vi "Populate Names.vi"(10 "Final  Output In":T1={"A-1,  1"="Main", "A-3,  2"="Main", "A-4, 3"="Recircirculation", "A-5, 4"="Scrubber", "A-7, 5"="Oxygen", "A-8, 6"="Vent", "B-1,  7"="Boost A", "B-3, 8"="Boost A", "B-4,  9"="Recircirculation", "B-5, 10"="Scrubber", "B-8, 11"="Vent", "C-1, 12"="Boost B", "C-3, 13"="Boost B", "C-4, 14"="Recircirculation", "C-5,  15"="Scrubber", "C-8, 16"="Vent", "D-1, 17"="Main", "D-3, 18"="Boost A", "D-4,  19"="Boost B", "D-5,  20"="Vent", "D-8,  21"="Vent 2", "B-7"="Oxygen", "C-7"="Oxygen", "D-7"="Oxygen", "A-1"=FALSE, "A-3"=FALSE, "A-4"=FALSE, "A-5"=FALSE, "A-7"=FALSE, "A-8"=FALSE, "B-1"=FALSE, "B-3"=FALSE, "B-4"=FALSE, "B-5"=FALSE, "B-7"=FALSE, "B-8"=FALSE, "C-1"=FALSE, "C-3"=FALSE, "C-4"=FALSE, "C-5"=FALSE, "C-7"=FALSE, "C-8"=FALSE, "D-1"=FALSE, "D-3"=FALSE, "D-4"=FALSE, "D-5"=FALSE, "D-7"=FALSE, "D-8"=FALSE}, 11 "Final Names":T2={"A-1, 1"="Main", "A-3, 2"="Main", "A-4, 3"="Recircirculation", "A-5, 4"="Scrubber", "A-7, 5"="Oxygen", "A-8, 6"="Vent", "B-1,  7"="Boost A", "B-3, 8"="Boost A", "B-4, 9"="Recircirculation", "B-5, 10"="Scrubber", "B-8, 11"="Vent", "C-1, 12"="Boost B", "C-3, 13"="Boost B", "C-4, 14"="Recircirculation", "C-5,  15"="Scrubber", "C-8, 16"="Vent", "D-1, 17"="Main", "D-3, 18"="Boost A", "D-4,  19"="Boost B", "D-5,  20"="Vent", "D-8,  21"="Vent 2"}) -> (3 "Final  Output Out":T1={"A-1,  1"="Main", "A-3,  2"="Main", "A-4, 3"="Recircirculation", "A-5, 4"="Scrubber", "A-7, 5"="Oxygen", "A-8, 6"="Vent", "B-1,  7"="Boost A", "B-3, 8"="Boost A", "B-4,  9"="Recircirculation", "B-5, 10"="Scrubber", "B-8, 11"="Vent", "C-1, 12"="Boost B", "C-3, 13"="Boost B", "C-4, 14"="Recircirculation", "C-5,  15"="Scrubber", "C-8, 16"="Vent", "D-1, 17"="Main", "D-3, 18"="Boost A", "D-4,  19"="Boost B", "D-5,  20"="Vent", "D-8,  21"="Vent 2", "B-7"="Oxygen", "C-7"="Oxygen", "D-7"="Oxygen", "A-1"=FALSE, "A-3"=FALSE, "A-4"=FALSE, "A-5"=FALSE, "A-7"=FALSE, "A-8"=FALSE, "B-1"=FALSE, "B-3"=FALSE, "B-4"=FALSE, "B-5"=FALSE, "B-7"=FALSE, "B-8"=FALSE, "C-1"=FALSE, "C-3"=FALSE, "C-4"=FALSE, "C-5"=FALSE, "C-7"=FALSE, "C-8"=FALSE, "D-1"=FALSE, "D-3"=FALSE, "D-4"=FALSE, "D-5"=FALSE, "D-7"=FALSE, "D-8"=FALSE})   [LabVIEW 2013]
doc: "Populate the names field on the boolean output indicator control."
uses:
  Type Defs/Named Final Output name list ordered.ctl
  Type Defs/Named Final Output name list with 02.ctl
panel:
  # "Channel A"
  # "Channel B"
  # "Channel C"
  # "Channel D"
  # "Channel A"
  # "Channel B"
  # "Channel C"
  # "Channel D"
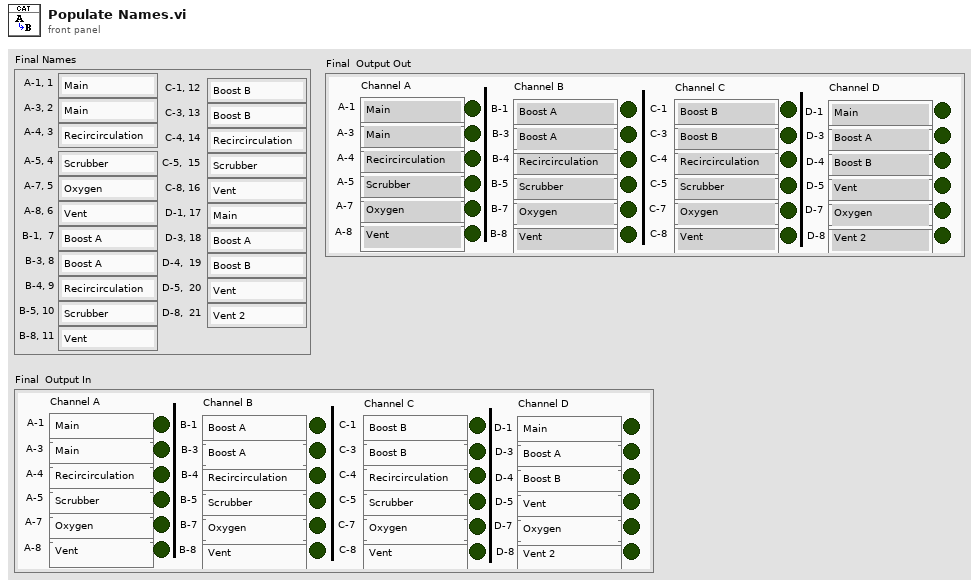
[diagram p1: front panel]
types:
  T1 = typedef "Named Final Output name list with 02.ctl" = cluster{"A-1,  1":string, "A-3,  2":string, "A-4, 3":string, "A-5, 4":string, "A-7, 5":string, "A-8, 6":string, "B-1,  7":string, "B-3, 8":string, "B-4,  9":string, "B-5, 10":string, "B-8, 11":string, "C-1, 12":string, "C-3, 13":string, "C-4, 14":string, "C-5,  15":string, "C-8, 16":string, "D-1, 17":string, "D-3, 18":string, "D-4,  19":string, "D-5,  20":string, "D-8,  21":string, "B-7":string, "C-7":string, "D-7":string, "A-1":bool, "A-3":bool, "A-4":bool, "A-5":bool, "A-7":bool, "A-8":bool, "B-1":bool, "B-3":bool, "B-4":bool, "B-5":bool, "B-7":bool, "B-8":bool, "C-1":bool, "C-3":bool, "C-4":bool, "C-5":bool, "C-7":bool, "C-8":bool, "D-1":bool, "D-3":bool, "D-4":bool, "D-5":bool, "D-7":bool, "D-8":bool}
  T2 = typedef "Named Final Output name list ordered.ctl" = cluster{"A-1, 1":string, "A-3, 2":string, "A-4, 3":string, "A-5, 4":string, "A-7, 5":string, "A-8, 6":string, "B-1,  7":string, "B-3, 8":string, "B-4, 9":string, "B-5, 10":string, "B-8, 11":string, "C-1, 12":string, "C-3, 13":string, "C-4, 14":string, "C-5,  15":string, "C-8, 16":string, "D-1, 17":string, "D-3, 18":string, "D-4,  19":string, "D-5,  20":string, "D-8,  21":string}
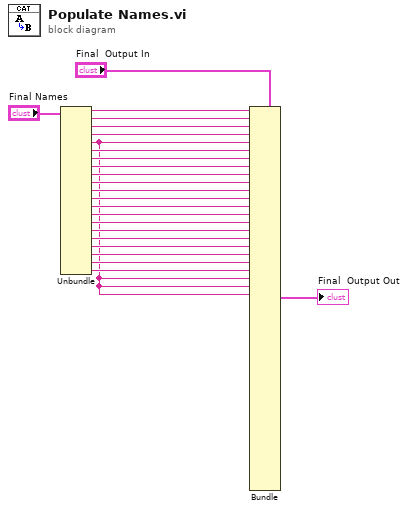
[diagram p0: block diagram]
diagram:
  n1 = Unbundle("Final Names") -> ("A-1, 1"=w22:string, "A-3, 2"=w21:string, "A-4, 3"=w20:string, "A-5, 4"=w19:string, "A-7, 5"=w2:string, "A-8, 6"=w18:string, "B-1,  7"=w17:string, "B-3, 8"=w16:string, "B-4, 9"=w15:string, "B-5, 10"=w14:string, "B-8, 11"=w12:string, "C-1, 12"=w13:string, "C-3, 13"=w11:string, "C-4, 14"=w10:string, "C-5,  15"=w9:string, "C-8, 16"=w8:string, "D-1, 17"=w7:string, "D-3, 18"=w6:string, "D-4,  19"=w5:string, "D-5,  20"=w4:string, "D-8,  21"=w3:string)
  n2 = Bundle(cluster="Final  Output In", "A-1,  1"=w22, "A-3,  2"=w21, "A-4, 3"=w20, "A-5, 4"=w19, "A-7, 5"=w2, "A-8, 6"=w18, "B-1,  7"=w17, "B-3, 8"=w16, "B-4,  9"=w15, "B-5, 10"=w14, "B-8, 11"=w12, "C-1, 12"=w13, "C-3, 13"=w11, "C-4, 14"=w10, "C-5,  15"=w9, "C-8, 16"=w8, "D-1, 17"=w7, "D-3, 18"=w6, "D-4,  19"=w5, "D-5,  20"=w4, "D-8,  21"=w3, "B-7"=w2, "C-7"=w2, "D-7"=w2) -> (→"Final  Output Out":T1)  [unwired: 24 in]
